vi "Main.vi"() -> ()   [LabVIEW 2020, in "DocTool.lvlib"]
uses:
  DocTool.lvlib
  TDefs/FP Items Properties Addendum.ctl
  TDefs/FP Items Properties.ctl
  TDefs/FP Item Properties.ctl
  TDefs/CopyTag.ctl
  TDefs/Single File Properties.ctl
  TDefs/Context.ctl
  Events/Events.ctl
  Events/UserEvent.ctl
  TDefs/State.ctl
  TDefs/States.ctl
  ce61f52e-de73-4afa-a1a4-5532dc3e8b5b.vi
  StateMachine.lvlib
panel:
  in  "Tab":enum32{"File Properties", "FP Items Properties"}(tab)
  in  "Write FP":bool
  in  "Copy_Desc":T1
  in  "Copy_HelpPath":T1
  in  "Copy_HelpTag":T1
  out "Progress":dbl(slide) scale=0.0..100.0 scale format="%#_4g"
  in  "File Properties":T2
  in  "PREV":bool
  in  "NEXT":bool
  in  "Read Folder":bool
  in  "Folder Path":path
  in  "SAVE":bool
  in  "Generate Help Tag":bool
  in  "Write":bool
  in  "Read File":bool
  out "VI Pic":picture
  out "VI Pic 2":picture
  in  "Connector Pane Terminals Only":bool
  in  "Tab Inputs":enum32{"Input", "More..."}(tab)
  in  "Inputs":T3
  in  "Input Addendum":T5
  in  "Tab Outputs":enum32{"Output", "More..."}(tab)
  in  "Outputs":T3
  in  "Output Addendum":T5
  in  "Mode":enum16{"All Items", "Selected Items"}(ring)
  in  "All":T1
  in  "Copy Descs to Tips":bool
  in  "Ignore Error Clusters":bool
  in  "Stop":bool
  # "%"
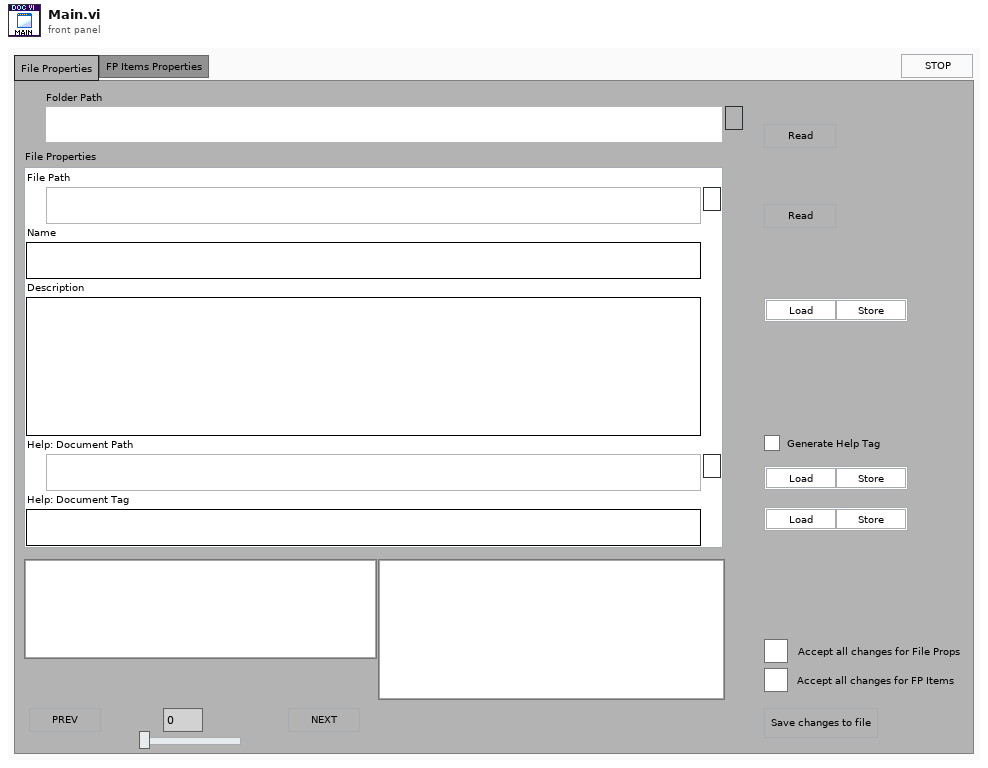
[diagram p1: front panel]
types:
  T1 = typedef "DocTool.lvlib/CopyTag.ctl" = cluster{"Load":bool, "Store":bool}
  T2 = typedef "DocTool.lvlib/Single File Properties.ctl" = cluster{"File Path":path, "Name":string, "Description":string, "Help: Document Path":path, "Help: Document Tag":string}
  T3 = typedef "DocTool.lvlib/FP Items Properties.ctl" = T4[]
  T4 = typedef "DocTool.lvlib/FP Item Properties.ctl" = cluster{"Sel":bool, "Idx":i32, "Name":string, "Description":string, "Tip":string, "Load Store":T1}
  T5 = typedef "DocTool.lvlib/FP Items Properties Addendum.ctl" = cluster{"Class Name":string[], "Class ID":dbl[]}
  T6 = typedef "DocTool.lvlib/Context.ctl" = cluster{"Events":T7, "States":cluster{"Current State":T9, "Next States":T10}, "General":cluster{"This VI":refnum<vi>, "Last Error":errorcluster}, "File":cluster{"Ref":refnum<vi>, "Props":T2, "Inputs":T3, "Outputs":T3, "Props Stored":T2, "Write":bool, "Write FP":bool, "Ignore Error Clusters":bool, "Copy Descs to Tips":bool, "CPTerminals Only":bool, "Generate Help Tag":bool}, "Progress":i32, "CtrlRefs":cluster{"File":cluster{"Properties":refnum<vi>, "Folder Path":refnum<vi>, "Read Folder":refnum<vi>, "Read File":refnum<vi>, "Path":refnum<vi>, "Help: Gen Tags":refnum<vi>, "Help: Doc Tag":refnum<vi>, "Help: Path":refnum<vi>}, "FP":cluster{"Inputs":refnum<vi>, "Outputs":refnum<vi>, "CP Terminals Only":refnum<vi>, "Ignore Error Clusters":refnum<vi>}}, "Folder":cluster{"Path":path, "File Paths":path[]}}
  T7 = typedef "StateMachine.lvlib/Events.ctl" = cluster{"Refnum":refnum<event-registration>, "Timeout":i32, "UserEvent":T8, "UserEvent Ref":refnum<user-event>}
  T8 = typedef "StateMachine.lvlib/UserEvent.ctl" = cluster{"ID":variant, "Data":variant}
  T9 = typedef "StateMachine.lvlib/State.ctl" = cluster{"ID":variant, "Data":variant}
  T10 = typedef "StateMachine.lvlib/States.ctl" = T9[]
  T11 = enum8{"Enabled", "Disabled", "Disabled and Grayed Out"}
  T12 = typedef "imagedata.ctl" = cluster{"image type":i32, "image depth":i32, "image":u8[], "mask":u8[], "colors":u32[], "Rectangle":cluster{"left":i16, "top":i16, "right":i16, "bottom":i16}}
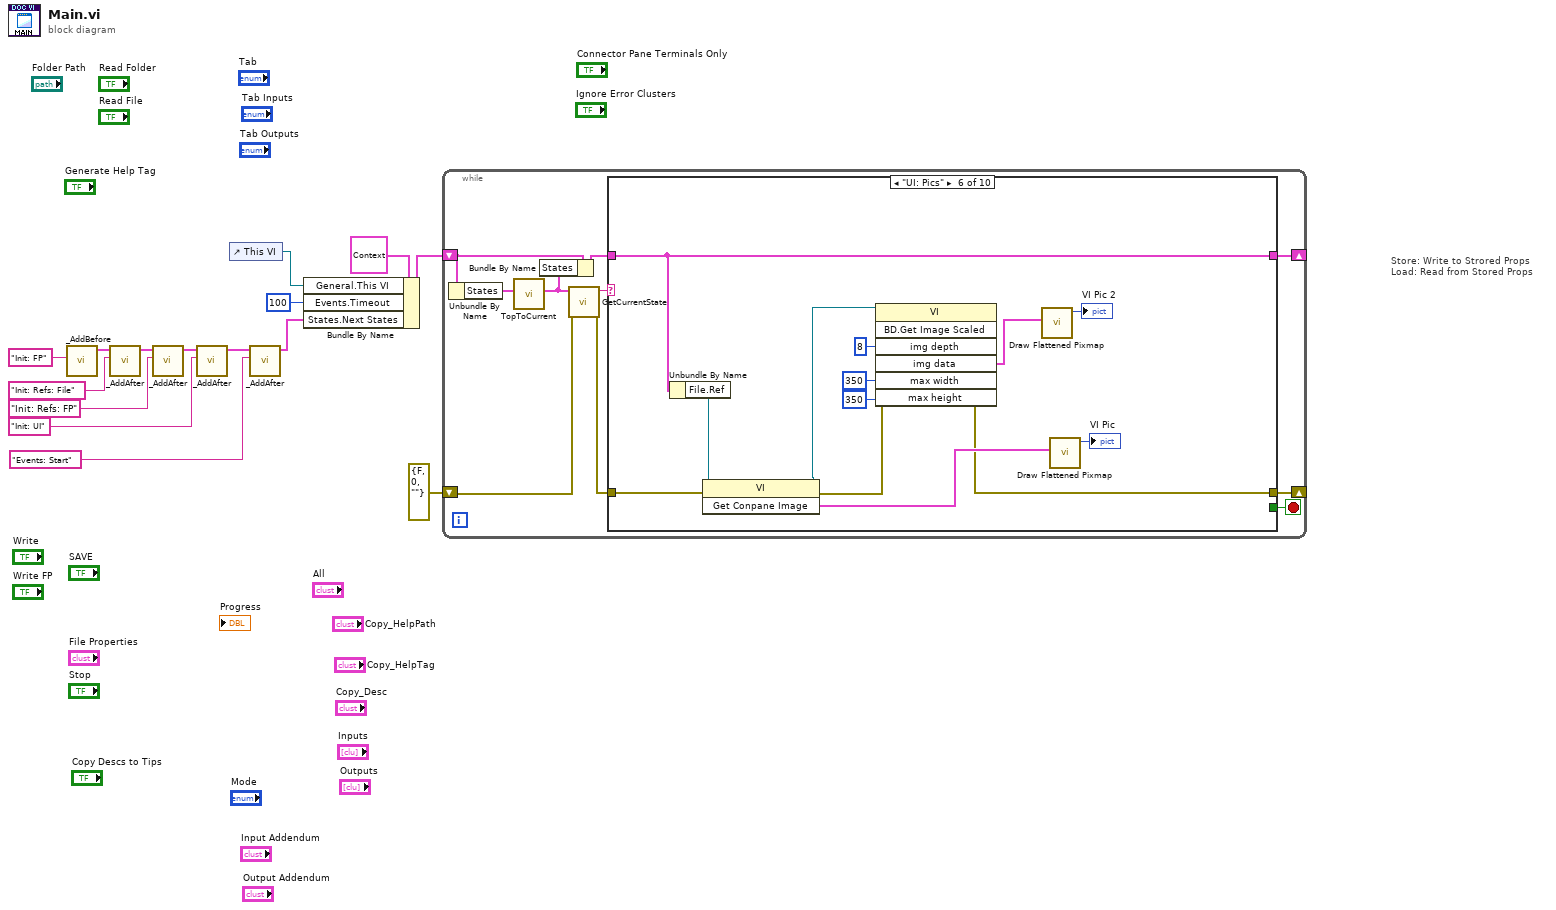
[diagram p0: block diagram]
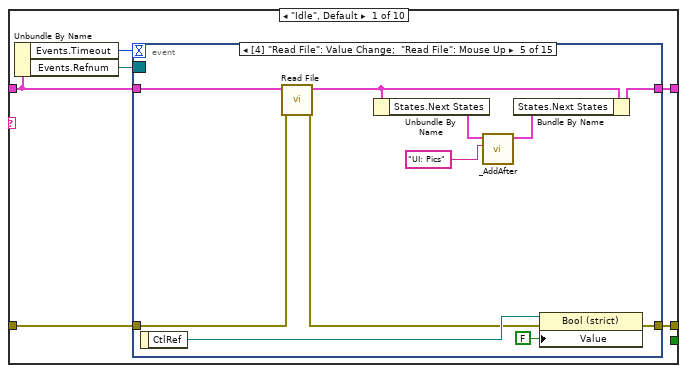
[diagram p2: hidden frame]
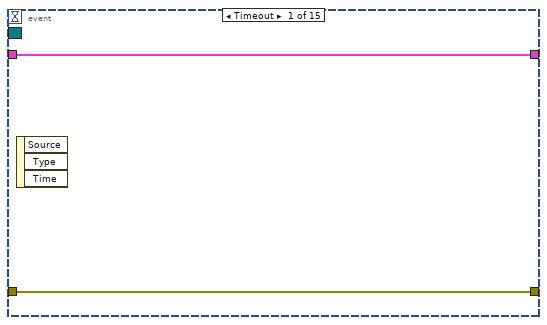
[diagram p3: hidden frame]
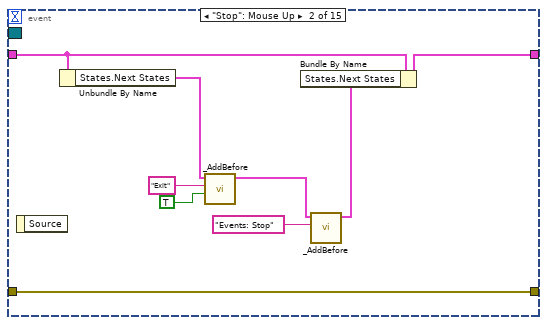
[diagram p4: hidden frame]
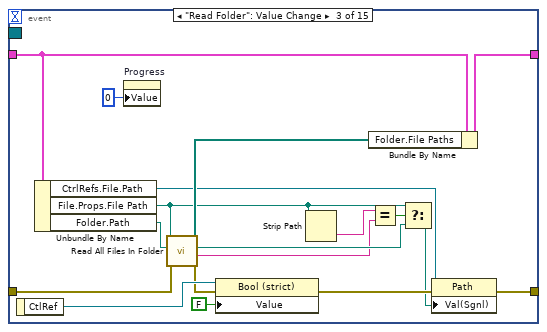
[diagram p5: hidden frame]
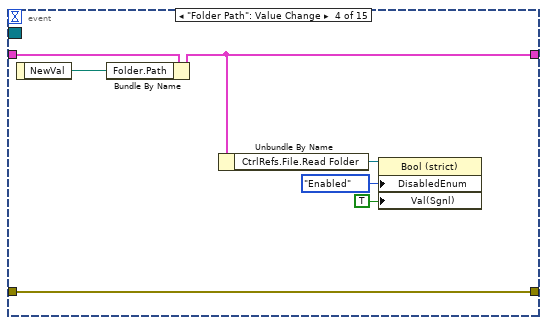
[diagram p6: hidden frame]
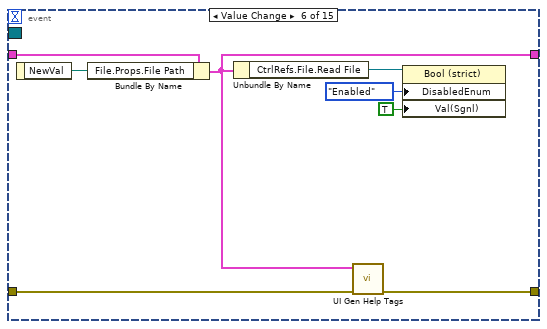
[diagram p7: hidden frame]
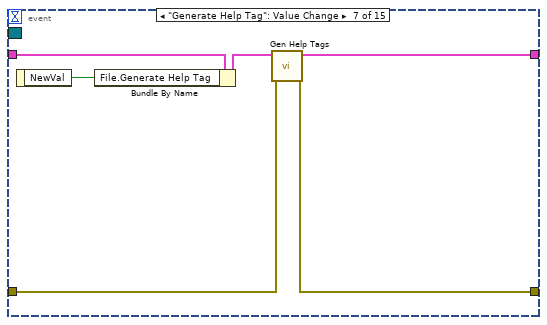
[diagram p8: hidden frame]
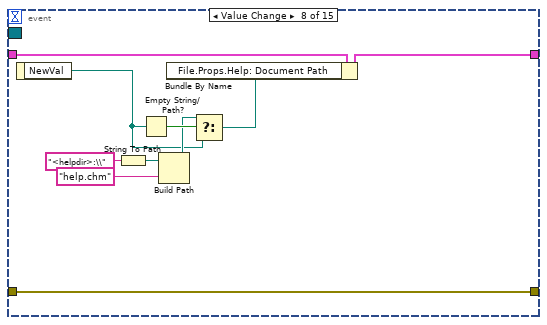
[diagram p9: hidden frame]
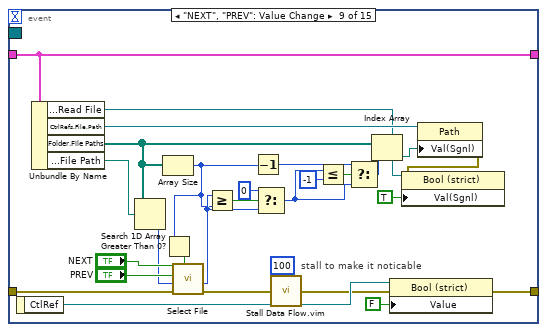
[diagram p10: hidden frame]
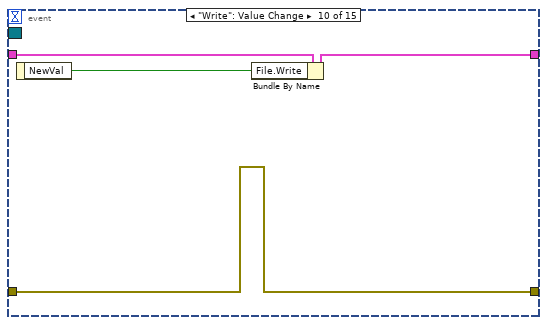
[diagram p11: hidden frame]
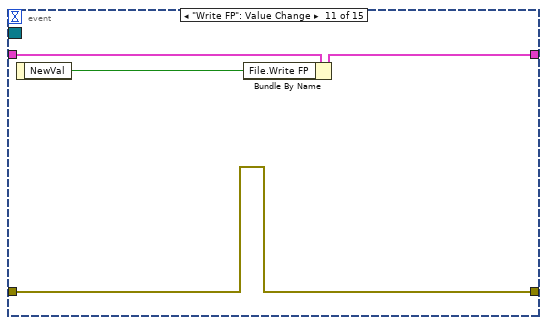
[diagram p12: hidden frame]
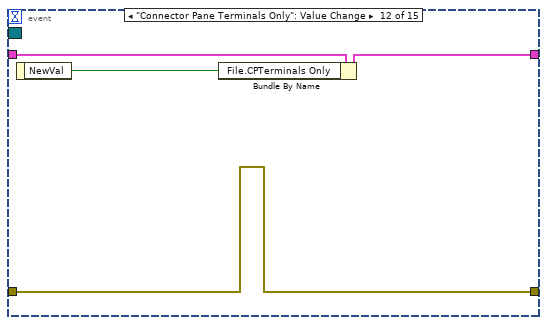
[diagram p13: hidden frame]
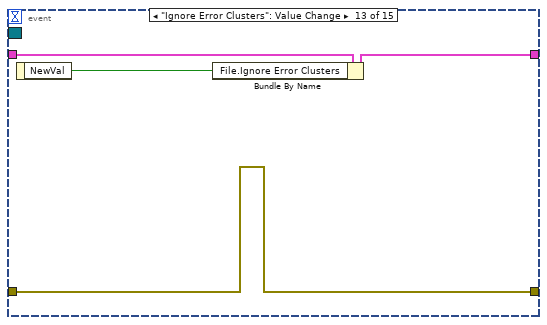
[diagram p14: hidden frame]
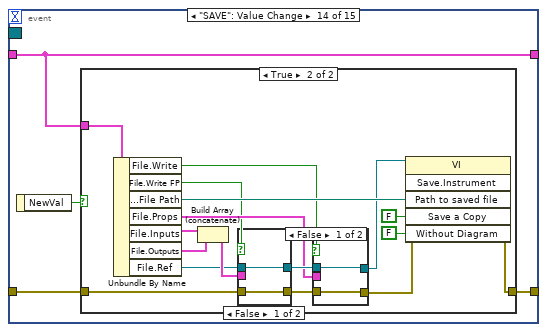
[diagram p15: hidden frame]
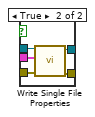
[diagram p17: hidden frame]
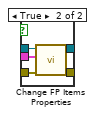
[diagram p18: hidden frame]
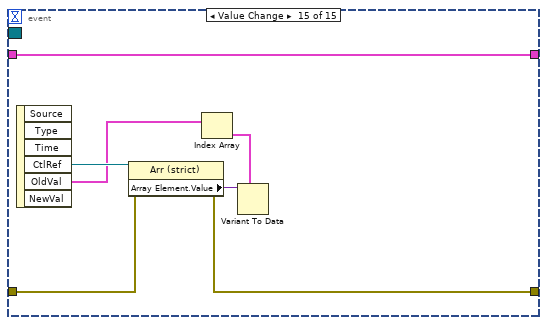
[diagram p19: hidden frame]
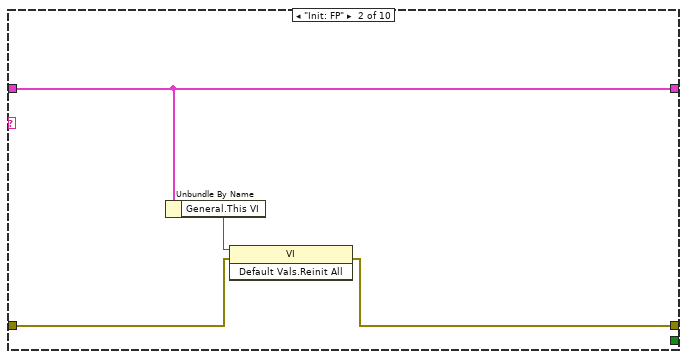
[diagram p20: hidden frame]
diagram:
  # "Store: Write to Strored Props\nLoad: Read from Stored Props"
  n1 = call "_AddBefore.vi"("ID"="Init: FP") -> ("Next States out"=w7:T10)  [unwired: 10 in]
  n2 = call "_AddAfter.vi"("ID"="Init: Refs: File", "Next States in"=w7) -> ("Next States out"=w5:T10)  [unwired: 9 in]
  n3 = call "_AddAfter.vi"("ID"="Init: Refs: FP", "Next States in"=w5) -> ("Next States out"=w3:T10)  [unwired: 9 in]
  n4 = call "_AddAfter.vi"("ID"="Init: UI", "Next States in"=w3) -> ("Next States out"=w2:T10)  [unwired: 9 in]
  n5 = control-ref of="This VI"() -> (w15:refnum<vi>)
  n6 = call "_AddAfter.vi"("ID"="Events: Start", "Next States in"=w2) -> ("Next States out"=w8:T10)  [unwired: 9 in]
  n7 = Bundle By Name(cluster=T6 {"Events"={"Refnum"=refnum, "Timeout"=0, "UserEvent"={"ID"=variant, "Data"=variant}, "UserEvent Ref"=refnum}, "States"={"Current State"={"ID"=variant, "Data"=variant}, "Next States"=[]}, "General"={"This VI"=refnum, "Last Error"={"status"=FALSE, "code"=0, "source"=""}}, "File"={"Ref"=refnum, "Props"={"File Path"=path "", "Name"="", "Description"="", "Help: Document Path"=path "", "Help: Document Tag"=""}, "Inputs"=[], "Outputs"=[], "Props Stored"={"File Path"=path "", "Name"="", "Description"="", "Help: Document Path"=path "", "Help: Document Tag"=""}, "Write"=FALSE, "Write FP"=FALSE, "Ignore Error Clusters"=FALSE, "Copy Descs to Tips"=FALSE, "CPTerminals Only"=FALSE, "Generate Help Tag"=FALSE}, "Progress"=0, "CtrlRefs"={"File"={"Properties"=refnum, "Folder Path"=refnum, "Read Folder"=refnum, "Read File"=refnum, "Path"=refnum, "Help: Gen Tags"=refnum, "Help: Doc Tag"=refnum, "Help: Path"=refnum}, "FP"={"Inputs"=refnum, "Outputs"=refnum, "CP Terminals Only"=refnum, "Ignore Error Clusters"=refnum}}, "Folder"={"Path"=path "", "File Paths"=[]}}, "General.This VI"=w15, "Events.Timeout"=100, "States.Next States"=w8) -> (w13:T6)
  n8 = while {
    shift-right: [w25] -> _
    shift-left: w13 -> [w21]
    shift-right: [w24] -> _
    shift-left: errorcluster {"status"=FALSE, "code"=0, "source"=""} ("error out") -> [w18]
    stop <- w23 stop-if-true
    n9 = Unbundle By Name(w21) -> ("States"=w16:cluster{"Current State":T9, "Next States":T10})
    n10 = call "TopToCurrent.vi"("States"=w16) -> ("States"=w17:cluster{"Current State":T9, "Next States":T10})  [unwired: 10 in]
    n11 = Bundle By Name(cluster=w21, "States"=w17) -> (w20:T6)
    n12 = call "GetCurrentState.vi"("error in (no error)"=w18, "States"=w17) -> ("error out"=w19:errorcluster, "Current State"=w22:string)  [unwired: 8 in]
    n13 = case shown="\"UI: Pics\"" w22 {
      tunnel: w20 -> [w27 w190 w204 w211 w223 w249 w252 w260 w264 w272]
      tunnel: [w26 w190 w202 w210 w226 w249 w252 w260 w264 w273] -> w25
      tunnel: w19 -> [w28 w192 w203 w207 w217 w250 w254 w256 w261 w269]
      tunnel: [w29 w191 w203 w207 w218 w239 errorcluster {"status"=FALSE, "code"=0, "source"=""} ("error out") w257 w265 w274] -> w24
      tunnel: [_ _ _ _ _ _ _ w255 _ _] -> w23
      frame "Idle", Default {
        n14 = Unbundle By Name(w27) -> ("Events.Timeout"=w30:i32, "Events.Refnum"=w31:refnum<event-registration>)
        n15 = event shown="[4] \"Read File\": Value Change;  \"Read File\": Mouse Up" {
          selector: w31 -> [_ _ _ _ _ _ _ _ _ _ _ _ _ _ _]
          dyn-events: _ -> [_ _ _ _ _ _ _ _ _ _ _ _ _ _ _]
          timeout: w30 -> [_ _ _ _ _ _ _ _ _ _ _ _ _ _ _]
          tunnel: [w33 w42 w57 w67 w74 w80 w89 w102 w124 w133 w137 w141 w145 w149 w187] -> w29
          tunnel: w28 -> [w33 w42 w60 w67 w78 w79 w90 w102 w130 w133 w137 w141 w145 w150 w188]
          tunnel: w27 -> [w32 w38 w58 w66 w77 w86 w92 w101 w127 w134 w138 w142 w146 w148 w186]
          tunnel: [w32 w39 w59 w64 w69 w81 w91 w100 w127 w132 w136 w140 w144 w148 w186] -> w26
          event Timeout {
            n16 = event-data() -> ()  [unwired: 1 in, 3 out]
          }
          event "Stop": Mouse Up {
            n17 = event-data() -> ()  [unwired: 1 in, 1 out]
            n18 = Unbundle By Name(w38) -> ("States.Next States"=w35:T10)
            n19 = call "_AddBefore.vi"("Data"=TRUE, "ID"="Exit", "Next States in"=w35) -> ("Next States out"=w36:T10)  [unwired: 8 in]
            n20 = call "_AddBefore.vi"("ID"="Events: Stop", "Next States in"=w36) -> ("Next States out"=w34:T10)  [unwired: 9 in]
            n21 = Bundle By Name(cluster=w38, "States.Next States"=w34) -> (w39:T6)
          }
          event "Read Folder": Value Change {
            n22 = event-data() -> ("CtlRef"=w53:refnum<vi>)  [unwired: 1 in]
            n23 = Unbundle By Name(w58) -> ("CtrlRefs.File.Path"=w49:refnum<vi>, "File.Props.File Path"=w43:path, "Folder.Path"=w56:path)
            n24 = property on="Progress" class="Slide (strict)"("Value"=0 ("Progress")) -> ()  [unwired: 2 in, 2 out]
            n25 = call "Read All Files In Folder.vi"("error in (no error)"=w60, "FolderPath"=w56, "Old File Path"=w43) -> ("error out"=w52:errorcluster, "File Name"=w44:string, "New File Path"=w45:path, "File Paths"=w55:path[])  [unwired: 5 in]
            n26 = property class="Bool (strict)"(reference=w53, error in=w52, "Value"=FALSE) -> (error out=w51:errorcluster)  [unwired: 1 out]
            n27 = Strip Path(path=w43) -> (name=w47:string)  [unwired: 1 out]
            n28 = Bundle By Name(cluster=w58, "Folder.File Paths"=w55) -> (w59:T6)
            n29 = Equal?(x=w47, y=w44) -> (x = y?=w46:bool)
            n30 = Select(t=w43, s=w46, f=w45) -> (s? t:f=w48:path)
            n31 = property on="Property Node" class="Path"(reference=w49, error in=w51, "Val(Sgnl)"=w48) -> (error out=w57:errorcluster)  [unwired: 1 out]
          }
          event "Folder Path": Value Change {
            n32 = event-data() -> ("NewVal"=w65:path)  [unwired: 1 in]
            n33 = Bundle By Name(cluster=w66, "Folder.Path"=w65) -> (w64:T6)
            n34 = Unbundle By Name(w64) -> ("CtrlRefs.File.Read Folder"=w63:refnum<vi>)
            n35 = property class="Bool (strict)"(reference=w63, "DisabledEnum"=T11."Enabled" ("Disabled"), "Val(Sgnl)"=TRUE ("Value (Signaling)")) -> ()  [unwired: 1 in, 2 out]
          }
          event "Read File": Value Change; "Read File": Mouse Up {
            n36 = event-data() -> ("CtlRef"=w75:refnum<vi>)  [unwired: 1 in]
            n37 = call "Read File.vi"("error in (no error)"=w78, "Context in"=w77) -> ("error out"=w73:errorcluster, "Context out"=w70:T6)  [unwired: 8 in]
            n38 = Unbundle By Name(w70) -> ("States.Next States"=w72:T10)
            n39 = call "_AddAfter.vi"("ID"="UI: Pics", "Next States in"=w72) -> ("Next States out"=w71:T10)  [unwired: 9 in]
            n40 = Bundle By Name(cluster=w70, "States.Next States"=w71) -> (w69:T6)
            n41 = property class="Bool (strict)"(reference=w75, error in=w73, "Value"=FALSE) -> (error out=w74:errorcluster)  [unwired: 1 out]
          }
          event Value Change {
            n42 = event-data() -> ("NewVal"=w85:path)  [unwired: 1 in]
            n43 = Bundle By Name(cluster=w86, "File.Props.File Path"=w85) -> (w81:T6)
            n44 = Unbundle By Name(w81) -> ("CtrlRefs.File.Read File"=w84:refnum<vi>)
            n45 = call "UI Gen Help Tags.vi"("error in (no error)"=w79, "Context"=w81) -> ("error out"=w80:errorcluster)  [unwired: 9 in]
            n46 = property class="Bool (strict)"(reference=w84, "DisabledEnum"=T11."Enabled" ("Disabled"), "Val(Sgnl)"=TRUE ("Value (Signaling)")) -> ()  [unwired: 1 in, 2 out]
          }
          event "Generate Help Tag": Value Change {
            n47 = event-data() -> ("NewVal"=w87:bool)  [unwired: 1 in]
            n48 = Bundle By Name(cluster=w92, "File.Generate Help Tag"=w87) -> (w88:T6)
            n49 = call "Gen Help Tags.vi"("error in (no error)"=w90, "Context in"=w88) -> ("error out"=w89:errorcluster, "Context out"=w91:T6)  [unwired: 8 in]
          }
          event Value Change {
            n50 = event-data() -> ("NewVal"=w94:path)  [unwired: 1 in]
            n51 = String To Path(string="<helpdir>:\\") -> (path=w97:path)
            n52 = Empty String/Path?(string/path=w94) -> (empty?=w96:bool)
            n53 = Build Path(base path=w97, name or relative path="help.chm") -> (appended path=w95:path)
            n54 = Select(t=w95, s=w96, f=w94) -> (s? t:f=w93:path)
            n55 = Bundle By Name(cluster=w101, "File.Props.Help: Document Path"=w93) -> (w100:T6)
          }
          event "NEXT", "PREV": Value Change {
            # "stall to make it noticable"
            n56 = event-data() -> ("CtlRef"=w126:refnum<vi>)  [unwired: 1 in]
            n57 = Unbundle By Name(w127) -> ("CtrlRefs.File.Read File"=w108:refnum<vi>, "CtrlRefs.File.Path"=w111:refnum<vi>, "Folder.File Paths"=w105:path[], "File.Props.File Path"=w110:path)
            n58 = Search 1D Array(1D array=w105, element=w110) -> (index of element=w109:i32)  [unwired: 1 in]
            n59 = Array Size(array=w105) -> (size(s)=w104:i32)
            n60 = Greater Than 0?(x=w104) -> (x > 0?=w103:bool)
            n61 = call "Select File.vi"("Files Found"=w103, "error in (no error)"=w130, "Current File in"=w109, "PREV"="PREV", "NEXT"="NEXT") -> ("error out"=w125:errorcluster, "Current File out"=w114:i32)  [unwired: 5 in]
            n62 = Greater Or Equal?(x=w114, y=w104) -> (x >= y?=w120:bool)
            n63 = Decrement(x=w104) -> (x-1=w116:i32)
            n64 = Select(t=0, s=w120, f=w114) -> (s? t:f=w115:i32)
            n65 = call "Stall Data Flow.vim"("value in"=w125, "milliseconds to wait"=u32 100) -> ("value out"=w122:errorcluster)  [unwired: 1 out]
            n66 = Less Or Equal?(x=w115, y=-1) -> (x <= y?=w117:bool)
            n67 = Select(t=w116, s=w117, f=w115) -> (s? t:f=w113:i32)
            n68 = Index Array(array=w105, index=w113) -> (element=w112:path)
            n69 = property class="Bool (strict)"(reference=w126, error in=w122, "Value"=FALSE) -> (error out=w124:errorcluster)  [unwired: 1 out]
            n70 = property class="Path"(reference=w111, "Val(Sgnl)"=w112) -> (error out=w106:errorcluster)  [unwired: 1 in, 1 out]
            n71 = property class="Bool (strict)"(reference=w108, error in=w106, "Val(Sgnl)"=TRUE ("Value (Signaling)")) -> ()  [unwired: 2 out]
          }
          event "Write": Value Change {
            n72 = event-data() -> ("NewVal"=w131:bool)  [unwired: 1 in]
            n73 = Bundle By Name(cluster=w134, "File.Write"=w131) -> (w132:T6)
          }
          event "Write FP": Value Change {
            n74 = event-data() -> ("NewVal"=w135:bool)  [unwired: 1 in]
            n75 = Bundle By Name(cluster=w138, "File.Write FP"=w135) -> (w136:T6)
          }
          event "Connector Pane Terminals Only": Value Change {
            n76 = event-data() -> ("NewVal"=w139:bool)  [unwired: 1 in]
            n77 = Bundle By Name(cluster=w142, "File.CPTerminals Only"=w139) -> (w140:T6)
          }
          event "Ignore Error Clusters": Value Change {
            n78 = event-data() -> ("NewVal"=w143:bool)  [unwired: 1 in]
            n79 = Bundle By Name(cluster=w146, "File.Ignore Error Clusters"=w143) -> (w144:T6)
          }
          event "SAVE": Value Change {
            n80 = event-data() -> ("NewVal"=w147:bool)  [unwired: 1 in]
            n81 = case shown="True" w147 {
              tunnel: w150 -> [w151 w156]
              tunnel: [w151 w165] -> w149
              tunnel: w148 -> [_ w164]
              frame False {
              }
              frame True {
                n82 = Unbundle By Name(w164) -> ("File.Write"=w152:bool, "File.Write FP"=w153:bool, "File.Props.File Path"=w166:path, "File.Props"=w158:T2, "File.Inputs"=w163:T3, "File.Outputs"=w162:T3, "File.Ref"=w157:refnum<vi>)
                n83 = Build Array (concatenate)(w163, w162) -> (w161:T3)
                n84 = case shown="False" w153 {
                  tunnel: w161 -> [_ w182]
                  tunnel: [w177 w181] -> w160
                  tunnel: w157 -> [w177 w180]
                  tunnel: w156 -> [w176 w179]
                  tunnel: [w176 w178] -> w155
                  frame False {
                  }
                  frame True {
                    n85 = call "Change FP Items Properties.vi"("error in (no error)"=w179, "Input + Output"=w182, "VI in"=w180) -> ("error out"=w178:errorcluster, "VI out"=w181:refnum<vi>)  [unwired: 7 in]
                  }
                }
                n86 = case shown="False" w152 {
                  tunnel: w160 -> [w169 w175]
                  tunnel: [w169 w174] -> w159
                  tunnel: w158 -> [_ w173]
                  tunnel: w155 -> [w170 w172]
                  tunnel: [w170 w171] -> w154
                  frame False {
                  }
                  frame True {
                    n87 = call "Write Single File Properties.vi"("error in (no error)"=w172, "File Properties in"=w173, "VI"=w175) -> ("error out"=w171:errorcluster, "VI out"=w174:refnum<vi>)  [unwired: 7 in]
                  }
                }
                n88 = invoke class="VI" method="Save.Instrument"(reference=w159, error in=w154, "Path to saved file"=w166, "Save a Copy"=FALSE, "Without Diagram"=FALSE) -> (error out=w165:errorcluster)  [unwired: 1 in, 5 out]
              }
            }
          }
          event Value Change {
            n89 = event-data() -> ("CtlRef"=w189:refnum<vi>, "OldVal"=w184:T3)  [unwired: 1 in, 4 out]
            n90 = property class="Arr (strict)"(reference=w189, error in=w188) -> (error out=w187:errorcluster, "Array Element.Value"=w185:variant)  [unwired: 1 out]
            n91 = Index Array(array=w184) -> (element=w183:T4)  [unwired: 1 in]
            n92 = Variant To Data(type=w183, Variant=w185) -> ()  [unwired: 1 in, 2 out]
          }
        }
      }
      frame "Init: FP" {
        n93 = Unbundle By Name(w190) -> ("General.This VI"=w193:refnum<vi>)
        n94 = invoke class="VI" method="Default Vals.Reinit All"(reference=w193, error in=w192) -> (error out=w191:errorcluster)  [unwired: 1 in, 2 out]
      }
      frame "Init: Refs: File" {
        n95 = control-ref of="Read Folder"() -> (w199:refnum<vi>)
        n96 = control-ref of="Read File"() -> (w198:refnum<vi>)
        n97 = control-ref of="Generate Help Tag"() -> (w196:refnum<vi>)
        n98 = control-ref of="File Properties"() -> (w201:refnum<vi>)
        n99 = control-ref of="Help: Document Tag"() -> (w195:refnum<vi>)
        n100 = control-ref of="Folder Path"() -> (w200:refnum<vi>)
        n101 = control-ref of="File Path"() -> (w197:refnum<vi>)
        n102 = control-ref of="Help: Document Path"() -> (w194:refnum<vi>)
        n103 = Bundle By Name(cluster=w204, "CtrlRefs.File.Properties"=w201, "CtrlRefs.File.Folder Path"=w200, "CtrlRefs.File.Read Folder"=w199, "CtrlRefs.File.Read File"=w198, "CtrlRefs.File.Path"=w197, "CtrlRefs.File.Help: Gen Tags"=w196, "CtrlRefs.File.Help: Doc Tag"=w195, "CtrlRefs.File.Help: Path"=w194) -> (w202:T6)
      }
      frame "Init: Refs: FP" {
        n104 = control-ref of="Connector Pane Terminals Only"() -> (w206:refnum<vi>)
        n105 = control-ref of="Ignore Error Clusters"() -> (w205:refnum<vi>)
        n106 = control-ref of="Inputs"() -> (w209:refnum<vi>)
        n107 = control-ref of="Outputs"() -> (w208:refnum<vi>)
        n108 = Bundle By Name(cluster=w211, "CtrlRefs.FP.Inputs"=w209, "CtrlRefs.FP.Outputs"=w208, "CtrlRefs.FP.CP Terminals Only"=w206, "CtrlRefs.FP.Ignore Error Clusters"=w205) -> (w210:T6)
      }
      frame "Init: UI" {
        n109 = Unbundle By Name(w223) -> ("CtrlRefs.File.Read Folder"=w230:refnum<vi>, "CtrlRefs.File.Read File"=w228:refnum<vi>)
        n110 = Unbundle By Name(w223) -> ("CtrlRefs.FP.CP Terminals Only"=w222:refnum<vi>, "CtrlRefs.FP.Ignore Error Clusters"=w221:refnum<vi>, "CtrlRefs.File.Help: Gen Tags"=w213:refnum<vi>)
        n111 = Build Array(w222, w221, w213) -> (w212:refnum<vi>[])
        n112 = Build Array (concatenate)(w230, w228, w212) -> (w229:refnum<vi>[])
        n113 = for {
          tunnel: w229 -> [w238] mode=indexing
          tunnel: w217 -> [w237]
          tunnel: [w236] -> w216 mode=indexing
          tunnel: T11."Disabled and Grayed Out" ("Disabled") -> [w235]
          n114 = property class="Bool (strict)"(reference=w238, error in=w237, "DisabledEnum"=w235) -> (error out=w236:errorcluster)  [unwired: 1 out]
        }
        n115 = for {
          tunnel: w212 -> [w234] mode=indexing
          tunnel: [w233] -> w219 mode=indexing
          tunnel: TRUE ("File.Copy Descs to Tips") -> [w232]
          tunnel: w217 -> [w231]
          n116 = property class="Bool (strict)"(reference=w234, error in=w231, "Value"=w232) -> (error out=w233:errorcluster)  [unwired: 1 out]
        }
        n117 = Merge Errors(w216, w219) -> (w218:errorcluster)
        n118 = Bundle By Name(cluster=w223, "File.Ignore Error Clusters"=TRUE, "File.Copy Descs to Tips"=TRUE, "File.CPTerminals Only"=TRUE, "File.Generate Help Tag"=TRUE) -> (w226:T6)
      }
      frame "UI: Pics" {
        n119 = Unbundle By Name(w249) -> ("File.Ref"=w248:refnum<vi>)
        n120 = invoke class="VI" method="Get Conpane Image"(reference=w248, error in=w250) -> (reference out=w241:refnum<vi>, error out=w240:errorcluster, "Get Conpane Image"=w251:T12)  [unwired: 1 in]
        n121 = invoke class="VI" method="BD.Get Image Scaled"(reference=w241, error in=w240, "img depth"=8 ("Image Depth"), "max width"=350 ("Maximum Width"), "max height"=350 ("Maximum Height")) -> (error out=w239:errorcluster, "img data"=w242:T12)  [unwired: 2 in, 5 out]
        n122 = call <vilib>:"Draw Flattened Pixmap.vi"("image data"=w242) -> ("new picture"=→"VI Pic 2":picture)  [unwired: 8 in]
        n123 = call <vilib>:"Draw Flattened Pixmap.vi"("image data"=w251) -> ("new picture"=→"VI Pic":picture)  [unwired: 8 in]
      }
      frame "Error" {
        n124 = call <vilib>:"Simple Error Handler.vi"("error in (no error)"=w254) -> ()  [unwired: 4 in, 5 out]
      }
      frame "Exit" {
        n125 = Unbundle By Name(w260) -> ("States.Current State.Data"=w259:variant)
        n126 = Variant To Data(error in=w256, type=FALSE, Variant=w259) -> (data=w255:bool, error out=w257:errorcluster)
      }
      frame "Events: Stop" {
        n127 = Unbundle By Name(w264) -> ("Events.Refnum"=w266:refnum<event-registration>, "Events.UserEvent Ref"=w263:refnum<user-event>)
        n128 = Destroy User Event(user event=w263, error in=w261) -> (error out=w262:errorcluster)
        n129 = Unregister For Events(event registration refnum=w266, error in=w262) -> (error out=w265:errorcluster)
      }
      frame "Events: Start" {
        n130 = Unbundle By Name(w272) -> ("Events.UserEvent"=w271:T8)
        n131 = Create User Event(user event datatype=w271, error in=w269) -> (user event=w267:refnum<user-event>, error out=w268:errorcluster)
        n132 = register-events(error in=w268, w267) -> (reference out=w270:refnum<event-registration>, error out=w274:errorcluster)  [unwired: 1 in]
        n133 = Bundle By Name(cluster=w272, "Events.UserEvent Ref"=w267, "Events.Refnum"=w270) -> (w273:T6)
      }
    }
  }
